vi "testAll.vi"(8 "error in (no error)":errorcluster) -> (0 "error out":errorcluster)   [LabVIEW 2018]
doc: "Test all public subVIs, exept runServer.vi."
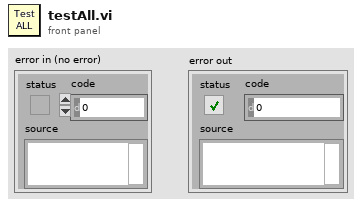
[diagram p1: front panel]
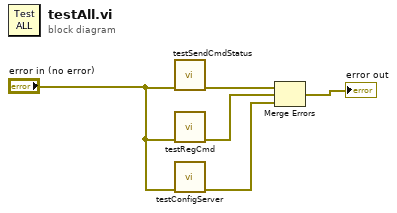
[diagram p0: block diagram]
diagram:
  n1 = call "testSendCmdStatus.vi"("error in (no error)"="error in (no error)") -> ("error out"=w4:errorcluster)  [unwired: 10 in]
  n2 = call "testRegCmd.vi"("error in (no error)"="error in (no error)") -> ("error out"=w2:errorcluster)  [unwired: 10 in]
  n3 = call "testConfigServer.vi"("error in (no error)"="error in (no error)") -> ("error out"=w1:errorcluster)  [unwired: 10 in]
  n4 = Merge Errors(w4, w2, w1) -> (→"error out":errorcluster)
